vi "Add Rx UDP Section and Status Channels.vi"(8 "error in":errorcluster, 10 "Rx UDP configuration":T7(array[cluster]) {"sapPorts"."Parameters"."Parameter"."encoding" items=["BNR", "BCD", "Discrete"]; "commPorts"."Parameters"."Parameter"."encoding" items=["BNR", "BCD", "Discrete"]; "Tx_UDP"."FilterMode" items=["FDX_RX_VL_FLT_DIS", "FDX_RX_VL_FLT_ENA ", "FDX_RX_VL_FLT_ENA_INV"]; "Tx_UDP"."VLBufSize" format="%.0x"; "Tx_UDP"."VerificationMode" items=["FDX_RX_VL_CHECK_ENA_DEFAULT"=65535, "FDX_RX_VL_CHECK_REDMAM"=16, "DX_RX_VL_CHECK_TRAFIC"=8, "FDX_RX_VL_CHECK_FRAMESIZE"=4, "FDX_RX_VL_CHECK_SNINTEG"=2, "FDX_RX_VL_CHECK_INVPAC"=1, "FDX_RX_VL_CHECK_DISA"=0]}, 11 "port ref":T8 format="%.0x") -> (0 "error out":errorcluster, 3 "port ref out":T8 format="%.0x")   [LabVIEW 2020, in "AIM ARINC 664 Scripting.lvlib"]
doc: "Add a Rx UDP page based on the Rx UDP configuration ."
uses:
  AIM ARINC 664 Scripting.lvlib
  <vilib>/NI VeriStand/Custom Device API/Custom Device Item Ref.ctl
  <vilib>/NI VeriStand/Custom Device API/Custom Device API.lvlib
  Import/_typedefs/frame_parameter_definition.ctl
  Import/AIM ARINC 664 Import.lvlib
  Import/_typedefs/rx_udp_setup.ctl
  Import/_typedefs/frame_parameter.ctl
  Import/_typedefs/port_rx_udp_comm.ctl
  Import/_typedefs/port_rx_udp_sap.ctl
  Shared/Encoding (Arinc664).ctl
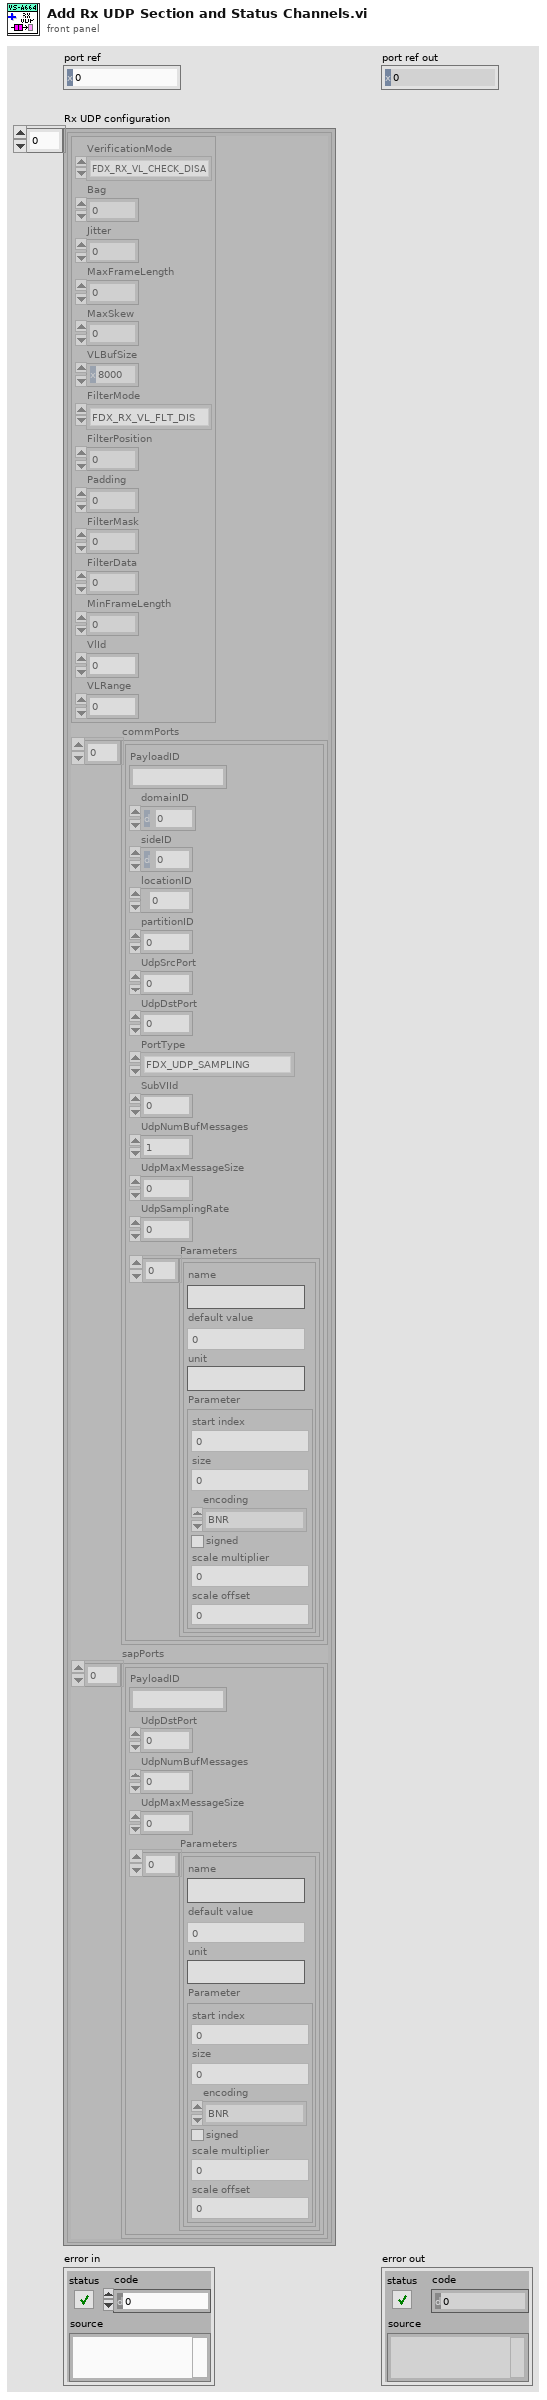
[diagram p1: front panel]
types:
  T1 = typedef "AIM ARINC 664 Import.lvlib/rx_udp_setup.ctl" = cluster{"VerificationMode":u32, "Bag":u32, "Jitter":u32, "MaxFrameLength":u32, "MaxSkew":u32, "VLBufSize":u32, "FilterMode":u32, "FilterPosition":u32, "Padding":u32, "FilterMask":u32, "FilterData":u32, "MinFrameLength":u32, "VlId":u16, "VLRange":u32}
  T2 = typedef "AIM ARINC 664 Import.lvlib/port_rx_udp_comm.ctl" = cluster{"PayloadID":string, "domainID":u8, "sideID":u8, "locationID":u8, "partitionID":u8, "UdpSrcPort":u16, "UdpDstPort":u16, "PortType":enum16{"FDX_UDP_SAMPLING", "FDX_UDP_QUEUING"}, "SubVIId":u32, "UdpNumBufMessages":u32, "UdpMaxMessageSize":u32, "UdpSamplingRate":u32, "Parameters":T3[]}
  T3 = typedef "AIM ARINC 664 Import.lvlib/frame_parameter.ctl" = cluster{"name":string, "default value":dbl, "unit":string, "Parameter":T4}
  T4 = typedef "AIM ARINC 664 Import.lvlib/frame_parameter_definition.ctl" = cluster{"start index":i32, "size":i32, "encoding":T5, "signed":bool, "scale multiplier":dbl, "scale offset":dbl}
  T5 = typedef "Encoding (Arinc664).ctl" = u16
  T6 = typedef "AIM ARINC 664 Import.lvlib/port_rx_udp_sap.ctl" = cluster{"PayloadID":string, "UdpDstPort":u16, "UdpNumBufMessages":u32, "UdpMaxMessageSize":u32, "Parameters":T3[]}
  T7 = cluster{"Tx_UDP":T1, "commPorts":T2[], "sapPorts":T6[]}[]
  T8 = typedef "Custom Device API.lvlib/Custom Device Item Ref.ctl" = u64
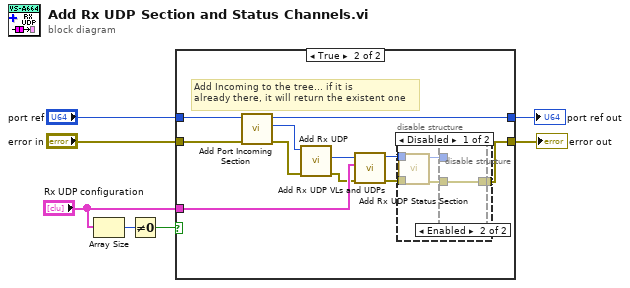
[diagram p0: block diagram]
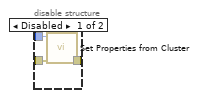
[diagram p3: hidden frame]
diagram:
  n1 = Array Size(array="Rx UDP configuration") -> (size(s)=w2:i32)
  n2 = Not Equal To 0?(x=w2) -> (x != 0?=w1:bool)
  n3 = case shown="True" w1 {
    tunnel: [w8 w20] -> w7
    tunnel: "error in" -> [w8 w19]
    tunnel: "port ref" -> [w9 w11]
    tunnel: [w9 w10] -> w4
    tunnel: "Rx UDP configuration" -> [_ w16]
    frame False {
    }
    frame True {
      # "Add Incoming to the tree... if it is \nalready there, it will return the existent one"
      n4 = call "Add Port Incoming Section.vi"("error in"=w19, "ports ref"=w11) -> ("error out"=w18:errorcluster, "incoming section ref out"=w17:T8, "ports ref out"=w10:T8)  [unwired: 7 in]
      n5 = call "Add Rx UDP.vi"("error in"=w18, "incoming ref"=w17) -> ("error out"=w13:errorcluster, "Rx UDP ref out"=w14:T8)  [unwired: 7 in, 1 out]
      n6 = call "Add Rx UDP VLs and UDPs.vi"("error in"=w13, "Rx UDP configuration"=w16, "Rx UDP ref"=w14) -> ("error out"=w12:errorcluster, "Rx UDP ref out"=w15:T8)  [unwired: 7 in]
      n7 = disable-structure shown="Disabled" {
        disable-tunnel: [w25 w30] -> w20
        disable-tunnel: w15 -> [w22 _]
        disable-tunnel: w12 -> [w21 w30]
        frame Disabled {
          n8 = call "Add Rx UDP Status Section.vi"("error in"=w21, "Rx UDP ref in"=w22) -> ("error out"=w24:errorcluster, "Rx UDP ref out"=w23:T8)  [unwired: 6 in, 2 out]
          n9 = disable-structure shown="Enabled" {
            disable-tunnel: [w28 w29] -> w25
            disable-tunnel: w24 -> [w27 w29]
            disable-tunnel: w23 -> [w26 _]
            frame Disabled {
              n10 = call "Set Properties from Cluster.vi"("error in"=w27, "item ref in"=w26) -> ("error out"=w28:errorcluster)  [unwired: 8 in, 1 out]
            }
            frame Enabled {
            }
          }
        }
        frame Enabled {
        }
      }
    }
  }
  "error out" <- w7
  "port ref out" <- w4
